vi "depth_servo.vi"(6 "Current depth":sgl[](array[numeric]), 9 "New command":bool, 10 "Goal position in":sgl[][](array[numeric]), 11 "Reset":bool) -> (3 "Goal position out":sgl[][](array[numeric]))   [LabVIEW 2013]
uses:
  utilities/labview/norm_vec_single.vi
  depth_servo_ui.vi
panel:
  out "Last goal position out":sgl[][](array[numeric])
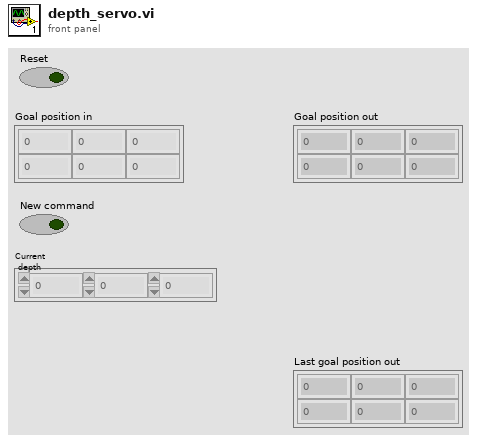
[diagram p1: front panel]
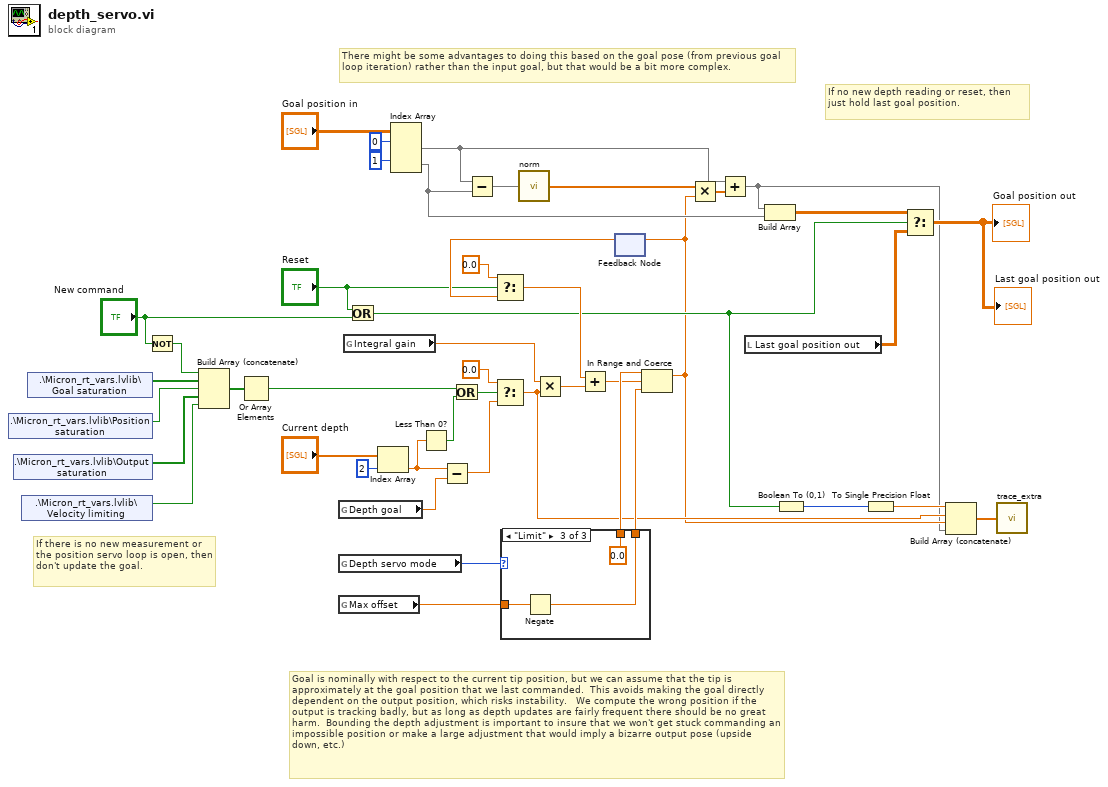
[diagram p0: block diagram]
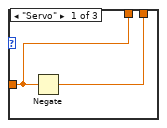
[diagram p2: hidden frame]
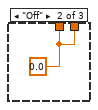
[diagram p3: hidden frame]
diagram:
  # "There might be some advantages to doing this based on the goal pose (from previous goal loop iteration) rather than the input goal, but that would be a bit more complex."
  # "If no new depth reading or reset, then just hold last goal position."
  # "If there is no new measurement or the position servo loop is open, then don't update the goal."
  # "Goal is nominally with respect to the current tip position, but we can assume that the tip is approximately at the goal position that we last commanded.  This avoids making the goal directly dependent on the output position, which risks instability.   We compute the wrong position if the output is tracking badly, but as long as depth updates are fairly frequent there should be no great harm.  Bounding the depth adjustment is important to insure that we won't get stuck commanding an impossible position or make a large adjustment that would imply a bizarre output pose (upside down, etc.)"
  n1 = shared-variable ".\\Micron_rt_vars.lvlib\\Position saturation"() -> (w29:bool)  [unwired: 1 in, 1 out]
  n2 = shared-variable ".\\Micron_rt_vars.lvlib\\Output saturation"() -> (w28:bool[])  [unwired: 1 in, 1 out]
  n3 = shared-variable ".\\Micron_rt_vars.lvlib\\Velocity limiting"() -> (w27:bool)  [unwired: 1 in, 1 out]
  n4 = shared-variable ".\\Micron_rt_vars.lvlib\\Goal saturation"() -> (w30:bool[])  [unwired: 1 in, 1 out]
  n5 = Not(x="New command") -> (.not. x?=w17:bool)
  n6 = Build Array (concatenate)(w17, w30, w29, w28, w27) -> (w26:bool[])
  n7 = Or Array Elements(Boolean array=w26) -> (logical OR=w13:bool)
  n8 = global read "depth_servo_ui.vi" "Depth goal"() -> (w41:sgl)
  n9 = global read "depth_servo_ui.vi" "Depth servo mode"() -> (w33:enum16{"Limit", "Servo", "Off"})
  n10 = global read "depth_servo_ui.vi" "Max offset"() -> (w38:sgl)
  n11 = global read "depth_servo_ui.vi" "Integral gain"() -> (w21:sgl)
  n12 = Or(x="Reset", y="New command") -> (x .or. y?=w7:bool)
  n13 = Index Array(array="Current depth", index=2) -> (element=w14:sgl)
  n14 = Index Array(array="Goal position in", index (row) #1=0 ("index (row)"), index (row) #2=1 ("index (row)")) -> (element #1=w36:sgl[], element #2=w31:sgl[])  [unwired: 2 in]
  n15 = Less Than 0?(x=w14) -> (x < 0?=w11:bool)
  n16 = Subtract(x=w14, y=w41) -> (x-y=w24:sgl)
  n17 = Or(x=w13, y=w11) -> (x .or. y?=w12:bool)
  n18 = Subtract(x=w36, y=w31) -> (x-y=w42:sgl[])
  n19 = Select(t=sgl 0.0, s=w12, f=w24) -> (s? t:f=w4:sgl)
  n20 = case shown="\"Limit\"" w33 {
    tunnel: w38 -> [w46 _ w50]
    tunnel: [w47 w48 w51] -> w37
    tunnel: [w46 w48 sgl 0.0 ("Max offset")] -> w32
    frame "Servo" {
      n21 = Negate(x=w46) -> (-x=w47:sgl)
    }
    frame "Off" {
      w48 = sgl 0.0 ("t")
    }
    frame "Limit" {
      n22 = Negate(x=w50) -> (-x=w51:sgl)
    }
  }
  n23 = call-poly "norm.vi"("vector"=w42) -> ("normalized vector"=w35:sgl[])  [unwired: 3 in, 1 out]
  n24 = Multiply(x=w21, y=w4) -> (x*y=w22:sgl)
  n25 = feedback #1() -> (w19:sgl)  [unwired: 1 in]
  n26 = Select(t=sgl 0.0, s="Reset", f=w19) -> (s? t:f=w18:sgl)
  n27 = Add(x=w18, y=w22) -> (x+y=w23:sgl)
  n28 = In Range and Coerce(upper limit=w32, x=w23, lower limit=w37) -> (coerced(x)=w3:sgl)  [unwired: 1 out]
  n29 = feedback-in #1(w3) -> ()
  n30 = Multiply(x=w35, y=w3) -> (x*y=w34:sgl[])
  n31 = Add(x=w36, y=w34) -> (x+y=w2:sgl[])
  n32 = local read "Last goal position out"() -> (w8:sgl[][])
  n33 = Build Array(w2, w31) -> (w10:sgl[][])
  n34 = Boolean To (0,1)(Boolean=w7) -> (0, 1=w6:i16)
  n35 = To Single Precision Float(number=w6) -> (single precision float=w5:sgl)
  n36 = Select(t=w10, s=w7, f=w8) -> (s? t:f=→"Last goal position out" →"Goal position out":sgl[][])
  n37 = Build Array (concatenate)(w5, w4, w3, w2) -> (w1:sgl[])
  n38 = call "trace_extra.vi"("Extra trace data"=w1) -> ()  [unwired: 1 in]
